vi "Outdent Subsquent Report.vi"(0 "report in":refnum<class "NI_report.lvclass">, 7 "level":i32, 11 "error in (no error)":errorcluster) -> (4 "report out":refnum<class "NI_report.lvclass">, 15 "error out":errorcluster)   [LabVIEW 2020, in "NI_report.lvclass"]
uses:
  NI_report.lvclass
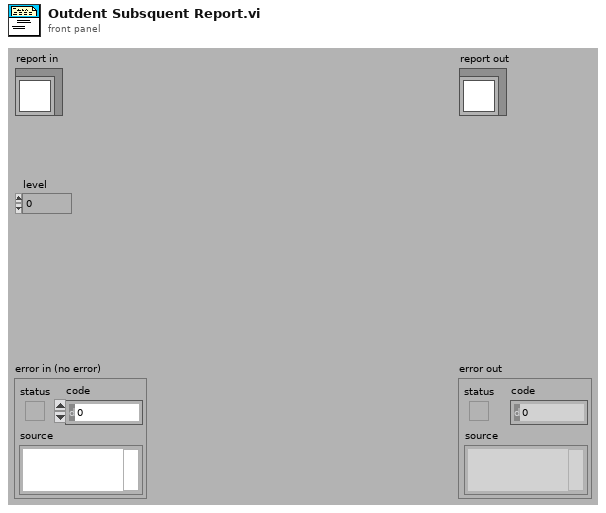
[diagram p1: front panel]
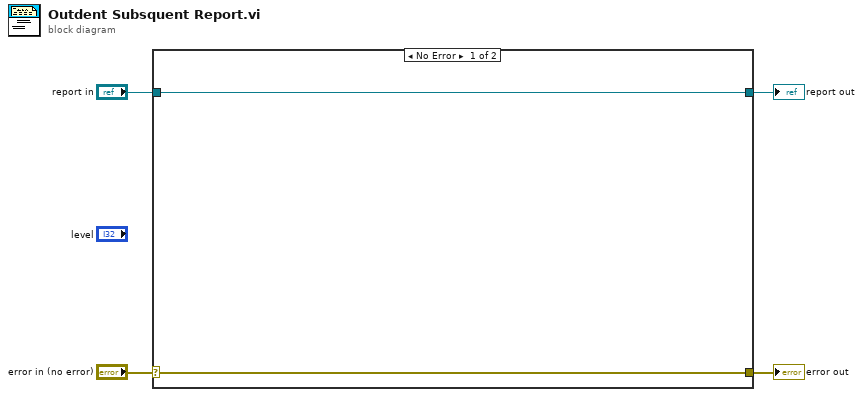
[diagram p0: block diagram]
diagram:
  n1 = case shown="No Error" "error in (no error)" {
    selector: "error in (no error)" -> [w5 w8]
    tunnel: [w5 w8] -> w3
    tunnel: [w6 w7] -> w1
    tunnel: "report in" -> [w6 w7]
    frame No Error {
    }
    frame Error {
    }
  }
  "error out" <- w3
  "report out" <- w1
